vi "TCPRouter ClientAPI Example 1.1.vi"() -> ()   [LabVIEW 2020]
uses:
  _addons/TCP-Router/ClientAPI/TcpRouter-Client.lvclass
panel:
  out "wait(ms)":u32
  out "Server Ready?":bool
  out "Response":string="DoA"
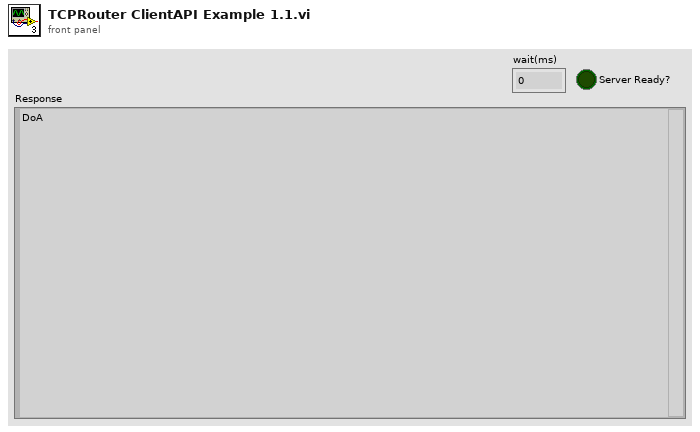
[diagram p1: front panel]
types:
  T1 = cluster{"IP Address":string, "Port":u16, "ConnectTMO":i32}
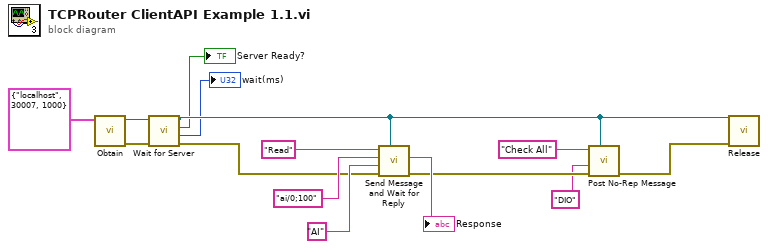
[diagram p0: block diagram]
diagram:
  n1 = call "Obtain.vi"("Connection"=T1 {"IP Address"="localhost", "Port"=30007, "ConnectTMO"=1000}) -> ("error out"=w6:errorcluster, "TcpRouter-Client out"=w5:refnum<class "TcpRouter-Client.lvclass">)  [unwired: 9 in]
  n2 = call "Wait for Server.vi"("error in (no error)"=w6, "TcpRouter-Client in"=w5) -> ("error out"=w4:errorcluster, "wait(ms)"=→"wait(ms)":u32, "Server Ready?"=→"Server Ready?":bool, "TcpRouter-Client out"=w3:refnum<class "TcpRouter-Client.lvclass">)  [unwired: 6 in]
  n3 = call "Send Message and Wait for Reply.vi"("TcpRouter-Client in"=w3, "error in (no error)"=w4, "Target Module"="AI", "Arguments (\"\")"="ai/0;100" ("State"), "State"="Read") -> ("error out"=w10:errorcluster, "Response"=→"Response":string)  [unwired: 5 in]
  n4 = call "Post No-Rep Message.vi"("TcpRouter-Client in"=w3, "error in (no error)"=w10, "Target Module"="DIO", "State"="Check All") -> ("error out"=w9:errorcluster)  [unwired: 7 in]
  n5 = call "Release.vi"("error in (no error)"=w9, "TcpRouter-Client in"=w3) -> ()  [unwired: 9 in, 1 out]
